vi "SRX_Send Point.vi"(7 "Point Array":T5[](array[typedef]), 8 "Error":errorcluster, 10 "Index":i32, 11 "CAN Talon SRX Ref":T1) -> (0 "Error Out":errorcluster, 1 "Last Point Out":bool, 2 "Next Index Out":i32, 3 "CAN Talon SRX Ref Out":T1, 5 "Buffer Full Out":bool)   [LabVIEW 2016]
uses:
  TypeDef/CLUSTER_Drive_Point Specification.ctl
  <vilib>/Rock Robotics/WPI/MotorControl/WPI_MotorControlDeviceRef.ctl
  <vilib>/Rock Robotics/WPI/MotorControl/WPI_MotorControlType.ctl
  <vilib>/Rock Robotics/SystemInterfaces/DIO/FPGA_DIOPWMChannel.ctl
  <vilib>/Rock Robotics/WPI/PWM/WPI_PWMDeadband.ctl
  <vilib>/Rock Robotics/WPI/ThirdParty/CanMotor/TalonSRX/WPI_CANTalonSRX_MotionProfileTrajectoryPt.ctl
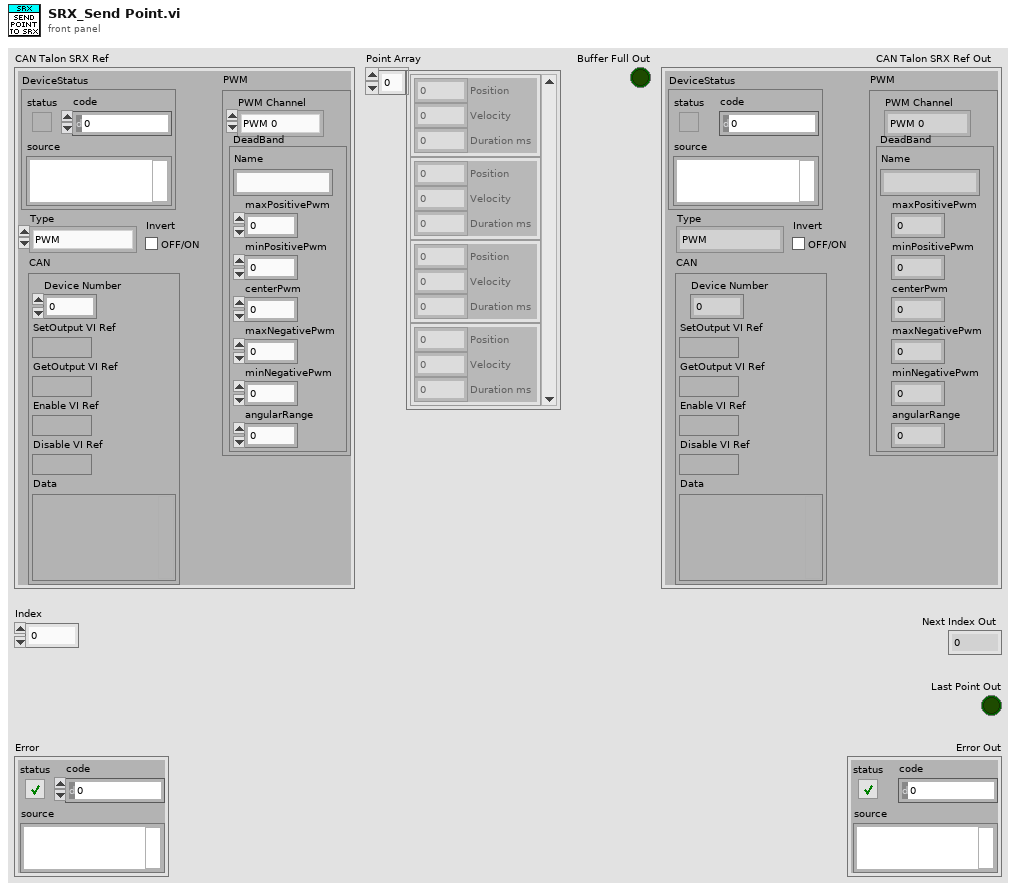
[diagram p1: front panel]
types:
  T1 = typedef "WPI_MotorControlDeviceRef.ctl" = cluster{"DeviceStatus":errorcluster, "Type":T2, "PWM":cluster{"PWM Channel":T3, "DeadBand":T4}, "CAN":cluster{"Device Number":u8, "SetOutput VI Ref":variant, "GetOutput VI Ref":variant, "Enable VI Ref":variant, "Disable VI Ref":variant, "Data":variant}, "Invert":bool}
  T2 = typedef "WPI_MotorControlType.ctl" = enum16{"PWM", "CAN"}
  T3 = typedef "FPGA_DIOPWMChannel.ctl" = enum8{"PWM 0", "PWM 1", "PWM 2", "PWM 3", "PWM 4", "PWM 5", "PWM 6", "PWM 7", "PWM 8", "PWM 9", "PWM MXP 0", "PWM MXP 1", "PWM MXP 2", "PWM MXP 3", "PWM MXP 4", "PWM MXP 5", "PWM MXP 6", "PWM MXP 7", "PWM MXP 8", "PWM MXP 9", "Invalid"}
  T4 = typedef "WPI_PWMDeadband.ctl" = cluster{"Name":string, "maxPositivePwm":i32, "minPositivePwm":i32, "centerPwm":i32, "maxNegativePwm":i32, "minNegativePwm":i32, "angularRange":u16}
  T5 = typedef "CLUSTER_Drive_Point Specification.ctl" = cluster{"Position":dbl, "Velocity":dbl, "Duration ms":u8}
  T6 = typedef "WPI_CANTalonSRX_MotionProfileTrajectoryPt.ctl" = cluster{"Duration Ms":u8, "Velocity":dbl, "Position":dbl, "Profile Slot Select":u8, "Is Last":bool, "Velocity Only":bool, "Zero Position":bool, "Compress Code":u8, "Same Velocity":i32, "Delta Position":i32, "Count":u8}
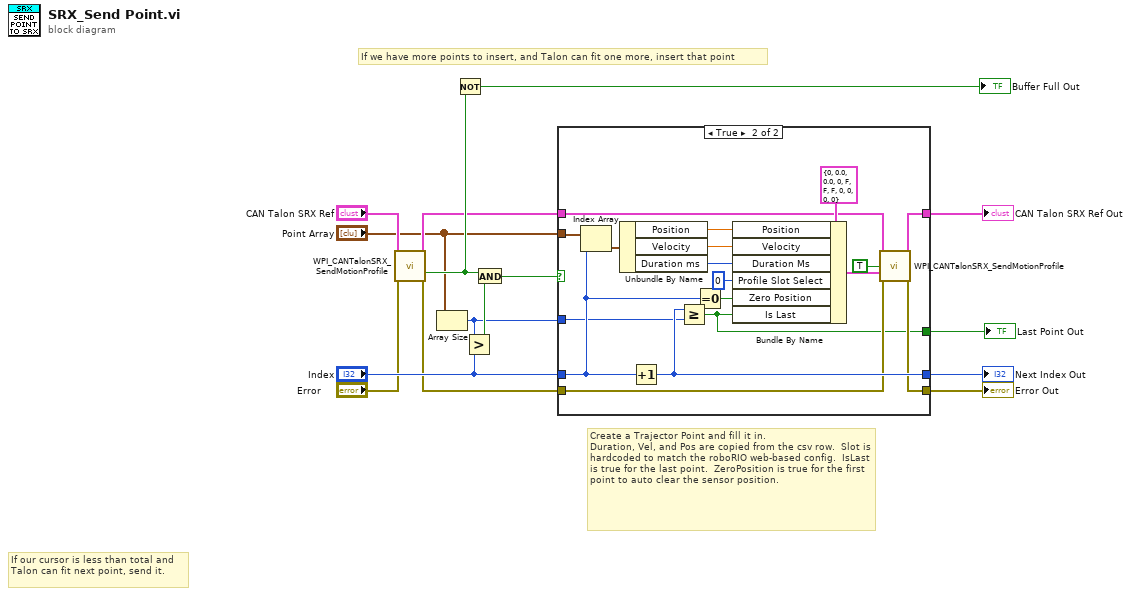
[diagram p0: block diagram]
diagram:
  # "Create a Trajector Point and fill it in.\nDuration, Vel, and Pos are copied from the csv row.  Slot is hardcoded to match the roboRIO web-based config.  IsLast is true for the last point.  ZeroPosition is true for the first point to auto clear the sensor position."
  # "If our cursor is less than total and Talon can fit next point, send it."
  # "If we have more points to insert, and Talon can fit one more, insert that point"
  n1 = call <vilib>:"WPI_CANTalonSRX_SendMotionProfile.vi"("CAN Talon SRX Ref"="CAN Talon SRX Ref", "Error"="Error") -> ("CAN Talon SRX Ref Out"=w13:T1, "Ready For Next Out"=w14:bool, "Error Out"=w7:errorcluster)  [unwired: 10 in, 1 out]
  n2 = Array Size(array="Point Array") -> (size(s)=w2:i32)
  n3 = Not(x=w14) -> (.not. x?=→"Buffer Full Out":bool)
  n4 = Greater?(x=w2, y="Index") -> (0:w15:bool)
  n5 = And(x=w14, y=w15) -> (x .and. y?=w11:bool)
  n6 = case shown="True" w11 {
    tunnel: "Point Array" -> [_ w35]
    tunnel: [w18 w30] -> w10
    tunnel: "Index" -> [w18 w31]
    tunnel: w2 -> [_ w28]
    tunnel: w13 -> [w16 w20]
    tunnel: w7 -> [w17 w23]
    tunnel: [w17 w22] -> w6
    tunnel: [_ w21] -> w5
    tunnel: [w16 w19] -> w4
    frame False {
    }
    frame True {
      n7 = Index Array(array=w35, index=w31) -> (element=w27:T5)
      n8 = Unbundle By Name(w27) -> ("Position"=w26:dbl, "Velocity"=w25:dbl, "Duration ms"=w24:u8)
      n9 = Increment(x=w31) -> (x+1=w30:i32)
      n10 = Greater Or Equal?(x=w30, y=w28) -> (x >= y?=w21:bool)
      n11 = Equal To 0?(x=w31) -> (x = 0?=w29:bool)
      n12 = Bundle By Name(cluster=T6 {"Duration Ms"=0, "Velocity"=0.0, "Position"=0.0, "Profile Slot Select"=0, "Is Last"=FALSE, "Velocity Only"=FALSE, "Zero Position"=FALSE, "Compress Code"=0, "Same Velocity"=0, "Delta Position"=0, "Count"=0} ("New Point"), "Position"=w26, "Velocity"=w25, "Duration Ms"=w24, "Profile Slot Select"=u8 0, "Zero Position"=w29, "Is Last"=w21) -> (w33:T6)
      n13 = call <vilib>:"WPI_CANTalonSRX_SendMotionProfile.vi"("CAN Talon SRX Ref"=w20, "Push"=TRUE, "New Point"=w33, "Error"=w23) -> ("CAN Talon SRX Ref Out"=w19:T1, "Error Out"=w22:errorcluster)  [unwired: 8 in, 2 out]
    }
  }
  "Next Index Out" <- w10
  "CAN Talon SRX Ref Out" <- w4
  "Error Out" <- w6
  "Last Point Out" <- w5
